vi "Autonomous Independent.vi"() -> ()   [LabVIEW 2013]
doc: "This VI is called when autonomous begins, and will automatically be terminated when autonomous ends. You can carry out timed or sensor driven robot movement independently without needing to return to the caller."
uses:
  <vilib>/Rock Robotics/WPI/DriverStation/WPI_DriverStationMatch Info.ctl
  Robot Global Data.vi
  <vilib>/Rock Robotics/WPI/RobotDrive/WPI_RobotDriveArcadeDrive_Standard(NoSaturation).vi
  <vilib>/Rock Robotics/WPI/RobotDrive/WPI_RobotDriveGetSetRefNum.vi
  <vilib>/Rock Robotics/WPI/Joystick/WPI_JoystickGetSetRefNum.vi
panel:
  in  "Match Info":T1={"Autonomous Elapsed Seconds"=0.0, "TeleOp Elapsed Seconds"=0.0, "Disabled Elapsed Seconds"=0.0, "Visited Autonomous"=FALSE, "Visited TeleOp"=FALSE, "Visited Disabled"=FALSE, "Autonomous Settings"={"Autonomous Style"=enum."Independent", "VI Refnum"=refnum}}
  in  "Scaling factor (V/in)":dbl=0.0098
  in  "Samples Per Second":dbl=1000.0
  in  "Average Bits":u8=3 max=15
  out "Current Movement, for debugging":T2 {"Y Joystick Value" scale=1.0..-1.0; "X Joystick Value" scale=-1.0..1.0}
  in  "Array of robot movements":T3(array[cluster]) {"Y Joystick Value" scale=1.0..-1.0; "X Joystick Value" scale=-1.0..1.0}
  # "Be sure to right-click and choose Data Operations>>Make Current Value default if you want to save the array values with the VI"
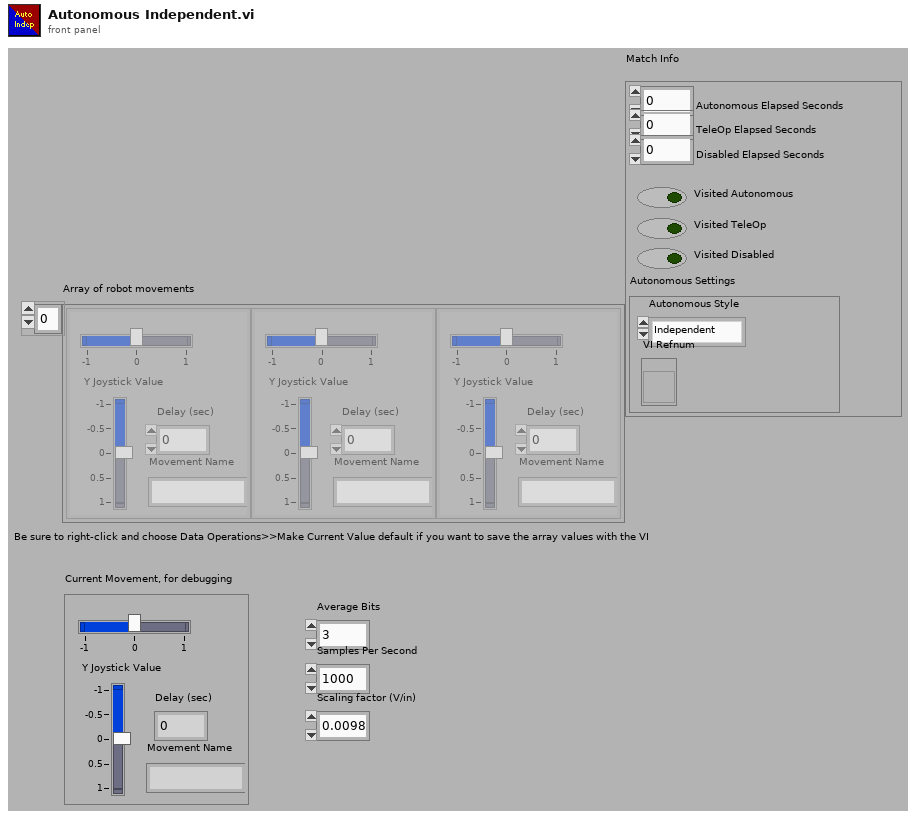
[diagram p1: front panel]
types:
  T1 = typedef "WPI_DriverStationMatch Info.ctl" = cluster{"Autonomous Elapsed Seconds":dbl, "TeleOp Elapsed Seconds":dbl, "Disabled Elapsed Seconds":dbl, "Visited Autonomous":bool, "Visited TeleOp":bool, "Visited Disabled":bool, "Autonomous Settings":cluster{"Autonomous Style":enum16{"Iterative", "Independent"}, "VI Refnum":refnum<vi>}}
  T2 = cluster{"X Joystick Value":dbl, "Y Joystick Value":dbl, "Delay (sec)":dbl, "Movement Name":string}
  T3 = cluster{"X Joystick Value":dbl, "Y Joystick Value":dbl, "Delay (sec)":dbl, "Movement Name":string}[]
  T4 = typedef "WPI_JoystickDevRef.ctl" = cluster{"Device":T5}
  T5 = typedef "WPI_JoystickDeviceEnum.ctl" = enum16{"USB 1", "USB 2", "USB 3", "USB 4", "Kinect 1", "Kinect 2"}
  T6 = cluster{"axis 1 (x)":dbl, "axis 2 (y)":dbl, "axis 3 (throttle)":dbl, "axis 4":dbl, "axis 5":dbl, "axis 6":dbl}
  T7 = typedef "WPI_RobotDriveDevRef.ctl" = cluster{"DevStatus":errorcluster, "Motors[]":T8[], "Square Inputs":bool, "Max Output":dbl, "Isochronous":bool}
  T8 = typedef "WPI_MotorControlDeviceRef.ctl" = cluster{"DeviceStatus":errorcluster, "Type":enum16{"PWM", "CAN"}, "PWM":cluster{"Digital Module":T9, "PWM Channel":T10, "DeadBand":T11}, "CAN":cluster{"Device Number":u8, "Control Mode":T12, "Semaphore":T13, "Max Vout":dbl}, "Invert":bool, "TransformRef":T14, "InvTransformRef":T14}
  T9 = typedef "FPGA_TypedefDigitalModule.ctl" = enum16{"Digital Module 1", "Digital Module 2"}
  T10 = typedef "FPGA_DIOPWMChannel.ctl" = enum8{"PWM 1", "PWM 2", "PWM 3", "PWM 4", "PWM 5", "PWM 6", "PWM 7", "PWM 8", "PWM 9", "PWM 10", "Invalid"}
  T11 = typedef "WPI_PWMDeadband.ctl" = cluster{"Name":string, "maxPositivePwm":i32, "minPositivePwm":i32, "centerPwm":i32, "maxNegativePwm":i32, "minNegativePwm":i32, "angularRange":u16}
  T12 = typedef "WPI_CANJaguar_ControlMode.ctl" = enum8{"Percent VBus", "Current", "Speed", "Position", "Voltage"}
  T13 = typedef "Semaphore RefNum" = refnum<k1>
  T14 = typedef "WPI_PWMTransform_ConPane.ctl" = refnum<vi>
  T15 = typedef "WPI_DigitalInputDevRef.ctl" = cluster{"DevStatus":errorcluster, "DIO Channel":T16, "Digital Module":T9}
  T16 = typedef "FPGA_DIOChannel.ctl" = enum8{"DIO 1", "DIO 2", "DIO 3", "DIO 4", "DIO 5", "DIO 6", "DIO 7", "DIO 8", "DIO 9", "DIO 10", "DIO 11", "DIO 12", "DIO 13", "DIO 14", "Invalid"}
  T17 = typedef "WPI_AnalogChannelDevRef.ctl" = cluster{"DevStatus":errorcluster, "Analog Module":T18, "Analog Channel":T19}
  T18 = typedef "FPGA_TypedefAnalogModule.ctl" = enum16{"Analog Module 1", "Analog Module 2"}
  T19 = typedef "FPGA_AIChannel.ctl" = enum8{"AI 1", "AI 2", "AI 3", "AI 4", "AI 5", "AI 6", "AI 7", "AI 8", "Invalid"}
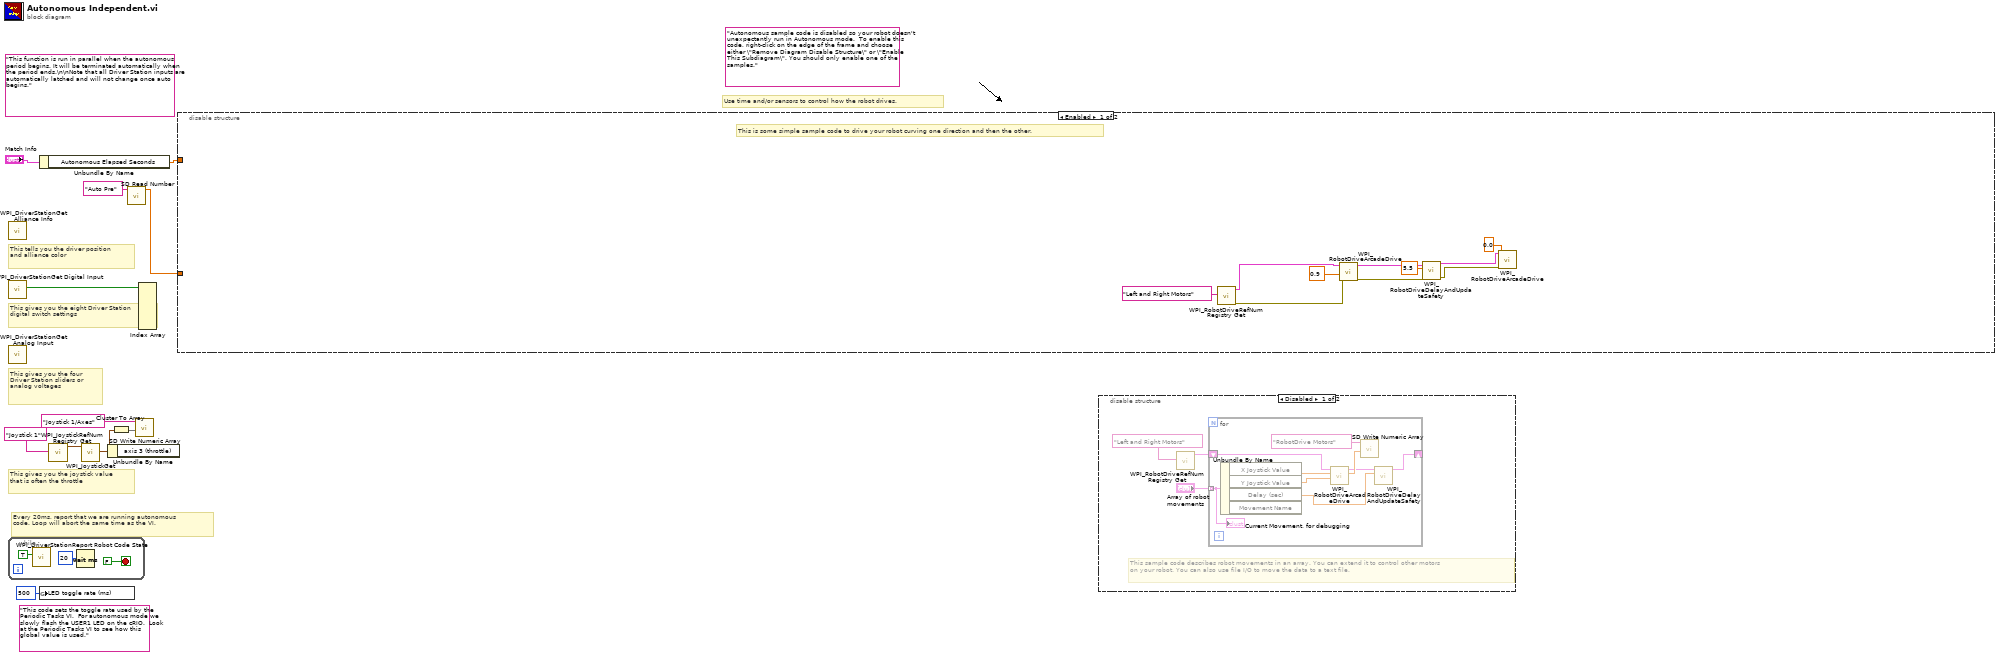
[diagram p0: block diagram]
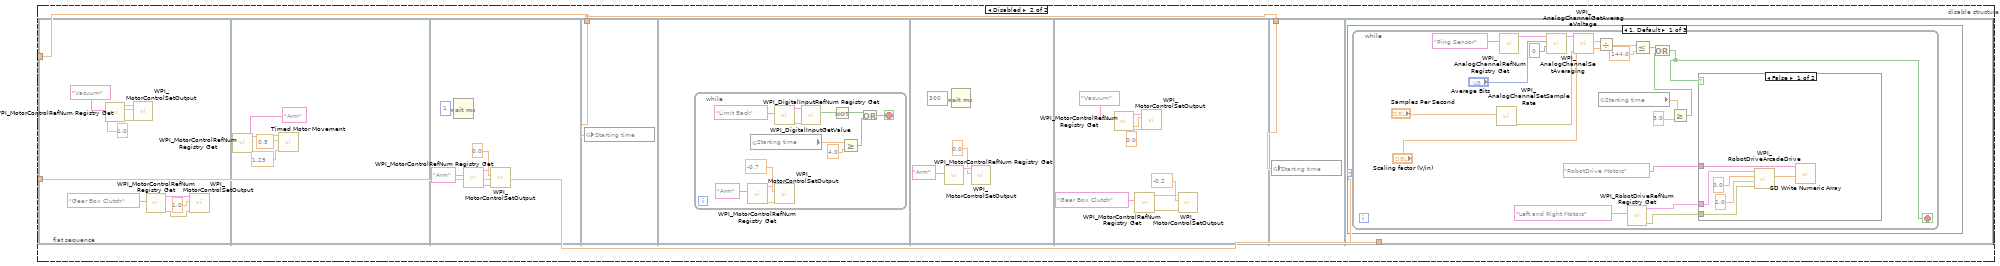
[diagram p3: hidden frame]
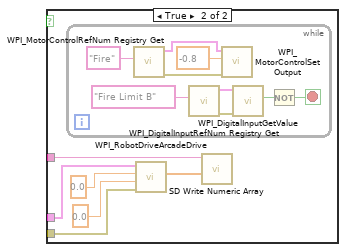
[diagram p4: hidden frame]
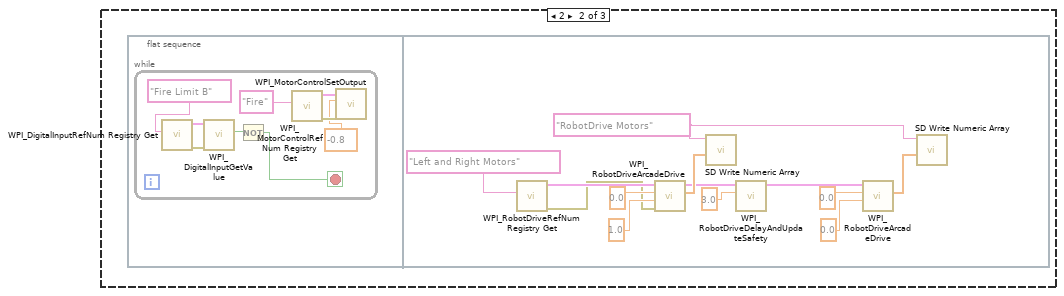
[diagram p5: hidden frame]
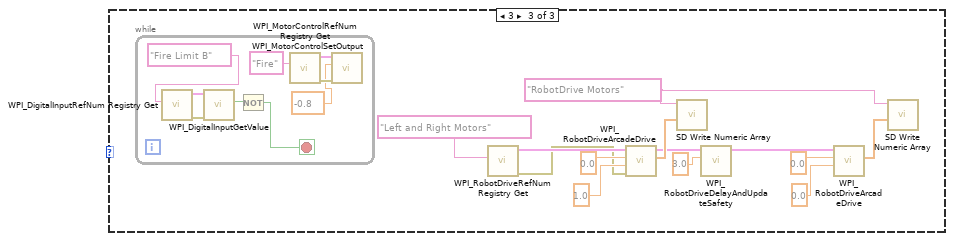
[diagram p6: hidden frame]
diagram:
  (unwired) "This code sets the toggle rate used by the Periodic Tasks VI.  For autonomous mode we slowly flash the USER1 LED on the cRIO.  Look at the Periodic Tasks VI to see how this global value is used."
  (unwired) "Autonomous sample code is disabled so your robot doesn't unexpectantly run in Autonomous mode.  To enable this code, right-click on the edge of the frame and choose either \"Remove Diagram Disable Structure\" or \"Enable This Subdiagram\". You should only enable one of the samples."
  (unwired) "This function is run in parallel when the autonomous period begins. It will be terminated automatically when the period ends.\n\nNote that all Driver Station inputs are automatically latched and will not change once auto begins."
  # "Every 20ms, report that we are running autonomous\ncode. Loop will abort the same time as the VI."
  # "This gives you the joystick value\nthat is often the throttle"
  # "Use time and/or sensors to control how the robot drives."
  # "This tells you the driver position\nand alliance color"
  # "This gives you the eight Driver Station\ndigital switch settings"
  # "This gives you the four\nDriver Station sliders or\nanalog voltages"
  n1 = while {
    stop <- FALSE stop-if-true
    n2 = call <vilib>:"WPI_DriverStationReport Robot Code State.vi"("Autonomous"=TRUE) -> ()  [unwired: 10 in, 1 out]
    n3 = Wait (ms)(milliseconds to wait=u32 20) -> ()  [unwired: 1 out]
  }
  n4 = call <vilib>:"WPI_DriverStationGet Alliance Info.vi"() -> ()  [unwired: 12 out]
  n5 = call <vilib>:"WPI_DriverStationGet Digital Input.vi"() -> ("Driver Station Digital Input (1-8)"=w11:bool[])  [unwired: 11 out]
  n6 = call <vilib>:"WPI_DriverStationGet Analog Input.vi"() -> ()  [unwired: 12 out]
  n7 = Unbundle By Name("Match Info") -> ("Autonomous Elapsed Seconds"=w1:dbl)
  n8 = global write "Robot Global Data.vi" "LED toggle rate (ms)"(u32 500 ("LED ms toggle rate")) -> ()
  n9 = call <vilib>:"WPI_JoystickRefNum Registry Get.vi"("refnum name"="Joystick 1") -> ("JoystickDevRef"=w9:T4)  [unwired: 1 in, 9 out]
  n10 = call <vilib>:"WPI_JoystickGet.vi"("JoystickDevRef"=w9) -> ("Axes"=w6:T6)  [unwired: 1 in, 5 out]
  n11 = Unbundle By Name(w6) -> ()  [unwired: 1 out]
  n12 = Cluster To Array(cluster=w6) -> (array=w7:dbl[])
  n13 = call <vilib>:"SD Read Number.vi"("Name"="Auto Pre") -> ("Numeric"=w3:dbl)  [unwired: 8 in, 2 out]
  n14 = call <vilib>:"SD Write Numeric Array.vi"("Numeric Array"=w7, "Name"="Joystick 1/Axes") -> ()  [unwired: 8 in, 2 out]
  n15 = Index Array(array=w11) -> ()  [unwired: 8 in, 8 out]
  n16 = disable-structure shown="Enabled" {
    disable-tunnel: w3 -> [_ w26]
    disable-tunnel: w1 -> [_ w25]
    frame Enabled {
      # "This is some simple sample code to drive your robot curving one direction and then the other."
      n17 = call <vilib>:"WPI_RobotDriveRefNum Registry Get.vi"("refnum name"="Left and Right Motors") -> ("error out"=w21:errorcluster, "RobotDriveDevRef"=w22:T7)  [unwired: 9 in]
      n18 = call-poly <vilib>:"WPI_RobotDriveArcadeDrive.vi"("error in (no error)"=w21, "Y axis value"=0.9, "RobotDriveDevRef"=w22) -> ("error out"=w19:errorcluster, "RobotDriveDevRef"=w20:T7)  [unwired: 6 in, 1 out]
      n19 = call <vilib>:"WPI_RobotDriveDelayAndUpdateSafety.vi"("error in (no error)"=w19, "Delay (s)"=5.5, "RobotDriveDevRef"=w20) -> ("error out"=w15:errorcluster, "RobotDriveDevRef 2"=w16:T7)  [unwired: 7 in]
      n20 = call-poly <vilib>:"WPI_RobotDriveArcadeDrive.vi"("error in (no error)"=w15, "Y axis value"=0.0, "RobotDriveDevRef"=w16) -> ()  [unwired: 6 in, 3 out]
    }
    frame Disabled {
      n21 = flat-sequence {
        tunnel: w25 -> [w44]
        tunnel: w25 -> [w70]
        tunnel: w26 -> [w71]
        frame #0 {
          n22 = call <vilib>:"WPI_MotorControlRefNum Registry Get.vi"("refnum name"="Vacuum") -> ("error out"=w32:errorcluster, "MotorControlDevRef"=w33:T8)  [unwired: 9 in]
          n23 = call <vilib>:"WPI_MotorControlSetOutput.vi"("error in (no error)"=w32, "Output"=1.0, "MotorControlDevRef"=w33) -> ()  [unwired: 6 in, 3 out]
          n24 = call <vilib>:"WPI_MotorControlRefNum Registry Get.vi"("refnum name"="Gear Box Clutch") -> ("error out"=w27:errorcluster, "MotorControlDevRef"=w30:T8)  [unwired: 9 in]
          n25 = call <vilib>:"WPI_MotorControlSetOutput.vi"("error in (no error)"=w27, "Output"=1.0 ("Numeric"), "MotorControlDevRef"=w30) -> ()  [unwired: 6 in, 3 out]
        }
        frame #1 {
          n26 = call <vilib>:"WPI_MotorControlRefNum Registry Get.vi"("refnum name"="Arm") -> ("MotorControlDevRef"=w35:T8)  [unwired: 9 in, 1 out]
          n27 = call "Timed Motor Movement.vi"("Seconds in"=1.25 ("Seconds to Turn"), "Power in"=0.5 ("Power"), "MotorControlDevRef"=w35) -> ()  [unwired: 4 in, 3 out]
        }
        frame #2 {
          n28 = Wait (ms)(milliseconds to wait=u32 1) -> ()  [unwired: 1 out]
          n29 = call <vilib>:"WPI_MotorControlRefNum Registry Get.vi"("refnum name"="Arm") -> ("error out"=w39:errorcluster, "MotorControlDevRef"=w41:T8)  [unwired: 9 in]
          n30 = call <vilib>:"WPI_MotorControlSetOutput.vi"("error in (no error)"=w39, "Output"=0.0, "MotorControlDevRef"=w41) -> ()  [unwired: 6 in, 3 out]
        }
        frame #3 {
          n31 = global write "Robot Global Data.vi" "Starting time"(w44) -> ()
        }
        frame #4 {
          n32 = while {
            stop <- w45 stop-if-true
            n33 = call <vilib>:"WPI_MotorControlRefNum Registry Get.vi"("refnum name"="Arm") -> ("error out"=w55:errorcluster, "MotorControlDevRef"=w56:T8)  [unwired: 9 in]
            n34 = global read "Robot Global Data.vi" "Starting time"() -> (w49:dbl)
            n35 = call <vilib>:"WPI_DigitalInputRefNum Registry Get.vi"("refnum name"="Limit Back") -> ("error out"=w51:errorcluster, "DigitalInputDevRef"=w52:T15)  [unwired: 9 in]
            n36 = call <vilib>:"WPI_MotorControlSetOutput.vi"("error in (no error)"=w55, "Output"=-0.7, "MotorControlDevRef"=w56) -> ()  [unwired: 6 in, 3 out]
            n37 = call <vilib>:"WPI_DigitalInputGetValue.vi"("error in (no error)"=w51, "DigitalInputDevRef"=w52) -> ("Value"=w50:bool)  [unwired: 7 in, 2 out]
            n38 = Not(x=w50) -> (.not. x?=w46:bool)
            n39 = Greater Or Equal?(x=w49, y=4.0) -> (x >= y?=w47:bool)
            n40 = Or(x=w46, y=w47) -> (x .or. y?=w45:bool)
          }
        }
        frame #5 {
          n41 = call <vilib>:"WPI_MotorControlRefNum Registry Get.vi"("refnum name"="Arm") -> ("MotorControlDevRef"=w61:T8)  [unwired: 9 in, 1 out]
          n42 = Wait (ms)(milliseconds to wait=u32 300) -> ()  [unwired: 1 out]
          n43 = call <vilib>:"WPI_MotorControlSetOutput.vi"("Output"=0.0, "MotorControlDevRef"=w61) -> ()  [unwired: 7 in, 3 out]
        }
        frame #6 {
          n44 = call <vilib>:"WPI_MotorControlRefNum Registry Get.vi"("refnum name"="Vacuum") -> ("error out"=w67:errorcluster, "MotorControlDevRef"=w68:T8)  [unwired: 9 in]
          n45 = call <vilib>:"WPI_MotorControlRefNum Registry Get.vi"("refnum name"="Gear Box Clutch") -> ("error out"=w62:errorcluster, "MotorControlDevRef"=w63:T8)  [unwired: 9 in]
          n46 = call <vilib>:"WPI_MotorControlSetOutput.vi"("error in (no error)"=w67, "Output"=0.0, "MotorControlDevRef"=w68) -> ()  [unwired: 6 in, 3 out]
          n47 = call <vilib>:"WPI_MotorControlSetOutput.vi"("error in (no error)"=w62, "Output"=-0.2 ("Numeric"), "MotorControlDevRef"=w63) -> ()  [unwired: 6 in, 3 out]
        }
        frame #7 {
          n48 = global write "Robot Global Data.vi" "Starting time"(w70) -> ()
        }
        frame #8 {
          n49 = case shown="1, Default" w71 {
            frame 1, Default {
              n50 = while {
                stop <- w75 stop-if-true
                n51 = call <vilib>:"WPI_AnalogChannelSetSampleRate.vi"("Samples Per Second"="Samples Per Second") -> ("error out"=w85:errorcluster)  [unwired: 3 in, 7 out]
                n52 = call <vilib>:"WPI_AnalogChannelRefNum Registry Get.vi"("refnum name"="Ping Sensor") -> ("AIDeviceRef"=w78:T17)  [unwired: 9 in, 1 out]
                n53 = call <vilib>:"WPI_AnalogChannelSetAveraging.vi"("OversampleBits"=u8 0, "AverageBits"="Average Bits", "AIDeviceRef"=w78) -> ("AIDeviceRef"=w84:T17)  [unwired: 1 in, 7 out]
                n54 = call <vilib>:"WPI_AnalogChannelGetAverageVoltage.vi"("error in (no error)"=w85, "AIDeviceRef"=w84) -> ("Voltage"=w83:dbl)  [unwired: 9 out]
                n55 = Divide(x=w83, y="Scaling factor (V/in)") -> (x/y=w86:dbl)
                n56 = global read "Robot Global Data.vi" "Starting time"() -> (w74:dbl)
                n57 = call <vilib>:"WPI_RobotDriveRefNum Registry Get.vi"("refnum name"="Left and Right Motors") -> ("error out"=w89:errorcluster, "RobotDriveDevRef"=w88:T7)  [unwired: 1 in, 8 out]
                n58 = Less Or Equal?(x=w86, y=144.0) -> (x <= y?=w76:bool)
                n59 = Greater Or Equal?(x=w74, y=3.0) -> (x >= y?=w72:bool)
                n60 = Or(x=w76, y=w72) -> (x .or. y?=w75:bool)
                n61 = case shown="False" w75 {
                  tunnel: w88 -> [w94 w100]
                  tunnel: w89 -> [w93 w99]
                  tunnel: "RobotDrive Motors" ("Name") -> [w92 w98]
                  frame False {
                    n62 = call-poly <vilib>:"WPI_RobotDriveArcadeDrive.vi"("error in (no error)"=w93, "Y axis value"=1.0 ("X axis value"), "X axis value"=0.0, "RobotDriveDevRef"=w94) -> ("Motor Values"=w95:dbl[])  [unwired: 7 out]
                    n63 = call <vilib>:"SD Write Numeric Array.vi"("Numeric Array"=w95, "Name"=w92) -> ()  [unwired: 8 in, 2 out]
                  }
                  frame True {
                    n64 = while {
                      stop <- w105 stop-if-true
                      n65 = call <vilib>:"WPI_MotorControlRefNum Registry Get.vi"("refnum name"="Fire") -> ("error out"=w109:errorcluster, "MotorControlDevRef"=w108:T8)  [unwired: 9 in]
                      n66 = call <vilib>:"WPI_DigitalInputRefNum Registry Get.vi"("refnum name"="Fire Limit B") -> ("error out"=w111:errorcluster, "DigitalInputDevRef"=w112:T15)  [unwired: 9 in]
                      n67 = call <vilib>:"WPI_MotorControlSetOutput.vi"("error in (no error)"=w109, "Output"=-0.8, "MotorControlDevRef"=w108) -> ()  [unwired: 6 in, 3 out]
                      n68 = call <vilib>:"WPI_DigitalInputGetValue.vi"("error in (no error)"=w111, "DigitalInputDevRef"=w112) -> ("Value"=w106:bool)  [unwired: 7 in, 2 out]
                      n69 = Not(x=w106) -> (.not. x?=w105:bool)
                    }
                    n70 = call-poly <vilib>:"WPI_RobotDriveArcadeDrive.vi"("error in (no error)"=w99, "Y axis value"=0.0 ("X axis value"), "X axis value"=0.0, "RobotDriveDevRef"=w100) -> ("Motor Values"=w101:dbl[])  [unwired: 7 out]
                    n71 = call <vilib>:"SD Write Numeric Array.vi"("Numeric Array"=w101, "Name"=w98) -> ()  [unwired: 8 in, 2 out]
                  }
                }
              }
            }
            frame 2 {
              n72 = flat-sequence {
                frame #0 {
                  n73 = while {
                    stop <- w114 stop-if-true
                    n74 = call <vilib>:"WPI_DigitalInputRefNum Registry Get.vi"("refnum name"="Fire Limit B") -> ("error out"=w120:errorcluster, "DigitalInputDevRef"=w121:T15)  [unwired: 9 in]
                    n75 = call <vilib>:"WPI_DigitalInputGetValue.vi"("error in (no error)"=w120, "DigitalInputDevRef"=w121) -> ("Value"=w115:bool)  [unwired: 7 in, 2 out]
                    n76 = Not(x=w115) -> (.not. x?=w114:bool)
                    n77 = call <vilib>:"WPI_MotorControlRefNum Registry Get.vi"("refnum name"="Fire") -> ("error out"=w118:errorcluster, "MotorControlDevRef"=w117:T8)  [unwired: 9 in]
                    n78 = call <vilib>:"WPI_MotorControlSetOutput.vi"("error in (no error)"=w118, "Output"=-0.8, "MotorControlDevRef"=w117) -> ()  [unwired: 6 in, 3 out]
                  }
                }
                frame #1 {
                  w134 = "RobotDrive Motors" ("Name")
                  n79 = call <vilib>:"WPI_RobotDriveRefNum Registry Get.vi"("refnum name"="Left and Right Motors") -> ("error out"=w122:errorcluster, "RobotDriveDevRef"=w131:T7)  [unwired: 1 in, 8 out]
                  n80 = call-poly <vilib>:"WPI_RobotDriveArcadeDrive.vi"("error in (no error)"=w122, "Y axis value"=1.0 ("X axis value"), "X axis value"=0.0, "RobotDriveDevRef"=w131) -> ("Motor Values"=w132:dbl[], "RobotDriveDevRef"=w127:T7)  [unwired: 6 out]
                  n81 = call <vilib>:"SD Write Numeric Array.vi"("Numeric Array"=w132, "Name"=w134) -> ()  [unwired: 8 in, 2 out]
                  n82 = call <vilib>:"WPI_RobotDriveDelayAndUpdateSafety.vi"("Delay (s)"=3.0, "RobotDriveDevRef"=w127) -> ("RobotDriveDevRef 2"=w128:T7)  [unwired: 8 in, 1 out]
                  n83 = call-poly <vilib>:"WPI_RobotDriveArcadeDrive.vi"("Y axis value"=0.0 ("X axis value"), "X axis value"=0.0, "RobotDriveDevRef"=w128) -> ("Motor Values"=w133:dbl[])  [unwired: 1 in, 7 out]
                  n84 = call <vilib>:"SD Write Numeric Array.vi"("Numeric Array"=w133, "Name"=w134) -> ()  [unwired: 8 in, 2 out]
                }
              }
            }
            frame 3 {
              w147 = "RobotDrive Motors" ("Name")
              n85 = while {
                stop <- w149 stop-if-true
                n86 = call <vilib>:"WPI_DigitalInputRefNum Registry Get.vi"("refnum name"="Fire Limit B") -> ("error out"=w155:errorcluster, "DigitalInputDevRef"=w156:T15)  [unwired: 9 in]
                n87 = call <vilib>:"WPI_DigitalInputGetValue.vi"("error in (no error)"=w155, "DigitalInputDevRef"=w156) -> ("Value"=w150:bool)  [unwired: 7 in, 2 out]
                n88 = Not(x=w150) -> (.not. x?=w149:bool)
                n89 = call <vilib>:"WPI_MotorControlRefNum Registry Get.vi"("refnum name"="Fire") -> ("error out"=w153:errorcluster, "MotorControlDevRef"=w152:T8)  [unwired: 9 in]
                n90 = call <vilib>:"WPI_MotorControlSetOutput.vi"("error in (no error)"=w153, "Output"=-0.8, "MotorControlDevRef"=w152) -> ()  [unwired: 6 in, 3 out]
              }
              n91 = call <vilib>:"WPI_RobotDriveRefNum Registry Get.vi"("refnum name"="Left and Right Motors") -> ("error out"=w135:errorcluster, "RobotDriveDevRef"=w144:T7)  [unwired: 1 in, 8 out]
              n92 = call-poly <vilib>:"WPI_RobotDriveArcadeDrive.vi"("error in (no error)"=w135, "Y axis value"=1.0 ("X axis value"), "X axis value"=0.0, "RobotDriveDevRef"=w144) -> ("Motor Values"=w145:dbl[], "RobotDriveDevRef"=w140:T7)  [unwired: 6 out]
              n93 = call <vilib>:"SD Write Numeric Array.vi"("Numeric Array"=w145, "Name"=w147) -> ()  [unwired: 8 in, 2 out]
              n94 = call <vilib>:"WPI_RobotDriveDelayAndUpdateSafety.vi"("Delay (s)"=3.0, "RobotDriveDevRef"=w140) -> ("RobotDriveDevRef 2"=w141:T7)  [unwired: 8 in, 1 out]
              n95 = call-poly <vilib>:"WPI_RobotDriveArcadeDrive.vi"("Y axis value"=0.0 ("X axis value"), "X axis value"=0.0, "RobotDriveDevRef"=w141) -> ("Motor Values"=w146:dbl[])  [unwired: 1 in, 7 out]
              n96 = call <vilib>:"SD Write Numeric Array.vi"("Numeric Array"=w146, "Name"=w147) -> ()  [unwired: 8 in, 2 out]
            }
          }
        }
      }
    }
  }
  n97 = disable-structure shown="Disabled" {
    frame Disabled {
      # "This sample code describes robot movements in an array. You can extend it to control other motors\non your robot. You can also use file I/O to move the data to a text file."
      n98 = call <vilib>:"WPI_RobotDriveRefNum Registry Get.vi"("refnum name"="Left and Right Motors") -> ("RobotDriveDevRef"=w158:T7)  [unwired: 1 in, 9 out]
      n99 = for {
        shift-right: [w164] -> _
        shift-left: w158 -> [w165]
        tunnel: "Array of robot movements" -> [w160] mode=indexing
        n100 = Unbundle By Name(w160) -> ("X Joystick Value"=w163:dbl, "Y Joystick Value"=w162:dbl, "Delay (sec)"=w161:dbl)  [unwired: 1 out]
        n101 = call-poly <vilib>:"WPI_RobotDriveArcadeDrive.vi"("Y axis value"=w162, "X axis value"=w163, "RobotDriveDevRef"=w165) -> ("Motor Values"=w167:dbl[], "RobotDriveDevRef"=w166:T7)  [unwired: 1 in, 6 out]
        n102 = call <vilib>:"SD Write Numeric Array.vi"("Numeric Array"=w167, "Name"="RobotDrive Motors") -> ()  [unwired: 8 in, 2 out]
        n103 = call <vilib>:"WPI_RobotDriveDelayAndUpdateSafety.vi"("Delay (s)"=w161, "RobotDriveDevRef"=w166) -> ("RobotDriveDevRef 2"=w164:T7)  [unwired: 8 in, 1 out]
        "Current Movement, for debugging" <- w160
      }
    }
    frame Enabled {
    }
  }
